vi "WeightingCheck.vi"() -> ()   [LabVIEW 2012]
uses:
  <vilib>/addons/database/Auxilliary.llb/DB Tools Cursor Type.ctl
  <vilib>/addons/database/Connection.llb/DB Tools Open Connec (Path).vi
  <vilib>/Utility/file.llb/Read From Spreadsheet File (string).vi
  <vilib>/addons/database/Connection.llb/Conn Execute.vi
  <vilib>/addons/database/Recordset.llb/Rec Fetch Integer Data (R).vi
  <vilib>/addons/database/Recordset.llb/Rec Destroy - Connection.vi
  <vilib>/Utility/file.llb/Write To Spreadsheet File (string).vi
  <vilib>/addons/database/NI_Database_API.lvlib
panel:
  out "error out":errorcluster
  out "filenames":string[](array[string])
  out "Wrong RC":bool
  out "STD Weight Check":bool
  out "ProdLine":bool
  out "Total Check":bool
  out "Pass Check":bool
  out "data":i32
  in  "Cluster":T1
  out "after substring":string
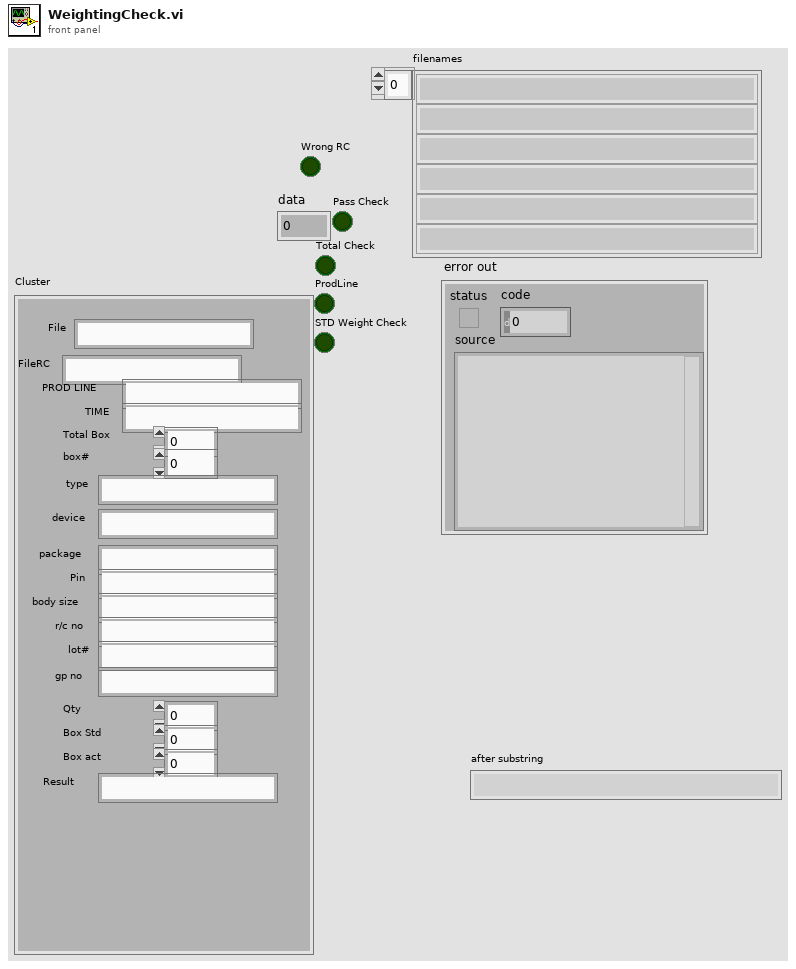
[diagram p1: front panel]
types:
  T1 = cluster{"File":string, "FileRC":string, "PROD LINE ":string, "TIME":string, "Total Box":dbl, "box#":dbl, "type":string, "device":string, "package":string, "Pin ":string, "body size":string, "r/c no":string, "lot#":string, "gp no":string, "Qty":dbl, "Box Std":dbl, "Box act":dbl, "Result":string}
  T2 = typedef "NI_Database_API.lvlib/DB Tools Cursor Type.ctl" = enum16{"forward-only", "keyset", "dynamic", "static"}
  T3 = typedef "NI_Database_API.lvlib/Conn ObjectReference.ctl" = refnum<k1>
  T4 = typedef "NI_Database_API.lvlib/Rec ObjectReference.ctl" = refnum<k1>
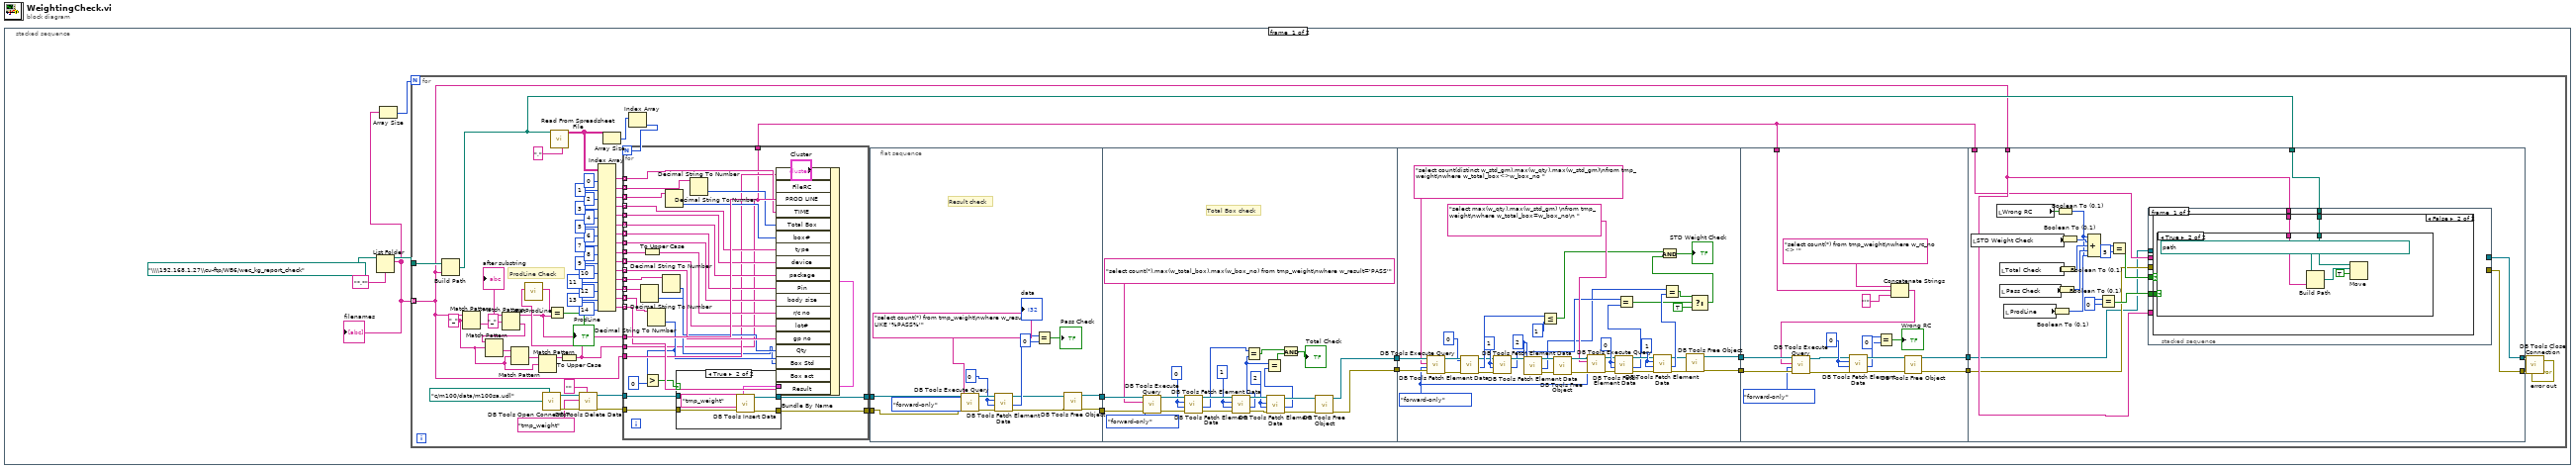
[diagram p0: block diagram]
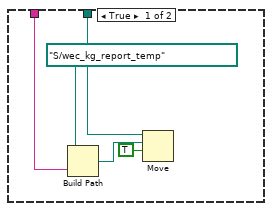
[diagram p2: hidden frame]
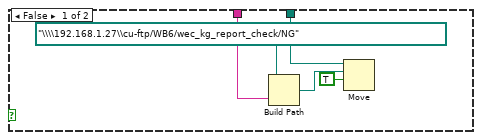
[diagram p3: hidden frame]
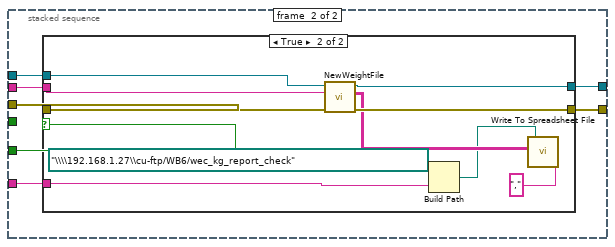
[diagram p4: hidden frame]
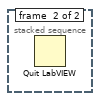
[diagram p7: hidden frame]
diagram:
  n1 = stacked-sequence {
    frame #0 {
      n2 = List Folder(path=path "\\\\192.168.1.27\\cu-ftp/WB6/wec_kg_report_check", pattern="*.*") -> (path out=w3:path, filenames=w1:string[])  [unwired: 2 in, 2 out]
      "filenames" <- w1
      n3 = Array Size(array=w1) -> (size(s)=w2:i32)
      n4 = for {
        N: w2 -> [_]
        tunnel: w3 -> [w56]
        tunnel: w1 -> [w10] mode=indexing
        w51 = "_" ("regular expression")
        # "ProdLine Check"
        n5 = Build Path(base path=w56, name or relative path=w10) -> (appended path=w11:path)
        n6 = Match Pattern(string=w10, regular expression=w51) -> (after substring=w54:string)  [unwired: 1 in, 3 out]
        "after substring" <- w54
        n7 = Match Pattern(string=w54, regular expression="_") -> (before substring=w19:string, after substring=w50:string)  [unwired: 1 in, 2 out]
        n8 = Match Pattern(string=w50, regular expression=w51) -> (after substring=w53:string)  [unwired: 1 in, 3 out]
        n9 = Match Pattern(string=w53, regular expression=w51) -> (after substring=w52:string)  [unwired: 1 in, 3 out]
        n10 = Match Pattern(string=w52, regular expression=w51) -> (before substring=w49:string)  [unwired: 1 in, 3 out]
        n11 = call-poly <vilib>:"DB Tools Open Connection.vi"("connection information"=path "c:/m100/data/m100sa.udl") -> ("error out"=w30:errorcluster, "connection reference"=w31:T3)  [unwired: 7 in]
        n12 = call-poly <vilib>:"Read From Spreadsheet File.vi"("delimiter (\\t)"="," ("delimiter (\\t)"), "file path (dialog if empty)"=w11) -> ("all rows"=w72:string[][])  [unwired: 5 in, 4 out]
        n13 = To Upper Case(1:w49) -> (0:w21:string)
        n14 = call "GetProdLine.vi"("Lotno"=w21) -> ("ProdLine"=w20:string)  [unwired: 10 in]
        n15 = Equal?(x=w20, y=w19) -> (x = y?=→"ProdLine":bool)
        n16 = call <vilib>:"DB Tools Delete Data.vi"("condition"="", "error in (no error)"=w30, "table"="tmp_weight", "connection reference"=w31) -> ("error out"=w28:errorcluster, "connection reference out"=w29:T3)  [unwired: 6 in]
        n17 = Index Array(array=w72, index (col) #1=0 ("disabled index (col)"), index (col) #2=1 ("index (col)"), index (col) #3=2 ("index (col)"), index (col) #4=3 ("index (col)"), index (col) #5=4 ("index (col)"), index (col) #6=5 ("index (col)"), index (col) #7=6 ("index (col)"), index (col) #8=7 ("index (col)"), index (col) #9=8 ("index (col)"), index (col) #10=9 ("index (col)"), index (col) #11=10 ("index (col)"), index (col) #12=11 ("index (col)"), index (col) #13=12 ("index (col)"), index (col) #14=13 ("index (col)"), index (col) #15=14 ("index (col)")) -> (element #1=w64:string[], element #2=w62:string[], element #3=w61:string[], element #4=w60:string[], element #5=w59:string[], element #6=w58:string[], element #7=w57:string[], element #8=w42:string[], element #9=w39:string[], element #10=w38:string[], element #11=w37:string[], element #12=w36:string[], element #13=w35:string[], element #14=w34:string[], element #15=w33:string[])  [unwired: 15 in]
        n18 = Array Size(array=w72) -> (size(s)=w73:i32[])
        n19 = Index Array(array=w73) -> (element=w63:i32)  [unwired: 1 in]
        n20 = for {
          N: w63 -> [_]
          tunnel: w64 -> [w258] mode=indexing
          tunnel: w62 -> [w261] mode=indexing
          tunnel: w61 -> [w256] mode=indexing
          tunnel: w60 -> [w254] mode=indexing
          tunnel: w59 -> [w253] mode=indexing
          tunnel: w58 -> [w252] mode=indexing
          tunnel: w57 -> [w251] mode=indexing
          tunnel: w42 -> [w250] mode=indexing
          tunnel: w39 -> [w262] mode=indexing
          tunnel: w38 -> [w248] mode=indexing
          tunnel: w37 -> [w247] mode=indexing
          tunnel: w36 -> [w246] mode=indexing
          tunnel: w35 -> [w244] mode=indexing
          tunnel: w34 -> [w243] mode=indexing
          tunnel: w33 -> [w242] mode=indexing
          tunnel: w21 -> [w231]
          tunnel: w10 -> [w241]
          tunnel: w19 -> [w259]
          tunnel: w29 -> [w240]
          tunnel: w28 -> [w239]
          tunnel: [w238] -> w25
          tunnel: [w237] -> w24
          tunnel: [w231] -> w7
          n21 = Decimal String To Number(string=w244) -> (number=w232:i32)  [unwired: 2 in, 1 out]
          n22 = To Upper Case(1:w262) -> (0:w249:string)
          n23 = Decimal String To Number(string=w243) -> (number=w235:i32)  [unwired: 2 in, 1 out]
          n24 = Greater?(x=w235, y=0) -> (0:w233:bool)
          n25 = Decimal String To Number(string=w246) -> (number=w245:i32)  [unwired: 2 in, 1 out]
          n26 = Decimal String To Number(string=w256) -> (number=w255:i32)  [unwired: 2 in, 1 out]
          n27 = Decimal String To Number(string=w261) -> (number=w257:i32)  [unwired: 2 in, 1 out]
          n28 = Bundle By Name(cluster="Cluster", "File"=w241, "FileRC"=w231, "PROD LINE"=w259, "TIME"=w258, "Total Box"=w257, "box#"=w255, "type"=w254, "device"=w253, "package"=w252, "Pin"=w251, "body size"=w250, "r/c no"=w249, "lot#"=w248, "gp no"=w247, "Qty"=w245, "Box Std"=w232, "Box act"=w235, "Result"=w242) -> (w236:T1)
          n29 = case shown="True" w233 {
            tunnel: w240 -> [w264 w270]
            tunnel: w239 -> [w263 w269]
            tunnel: [w264 w268] -> w238
            tunnel: [w263 w267] -> w237
            tunnel: w236 -> [_ w266]
            frame False {
            }
            frame True {
              n30 = call <vilib>:"DB Tools Insert Data.vi"("data"=w266, "error in (no error)"=w269, "table"="tmp_weight", "connection reference"=w270) -> ("error out"=w267:errorcluster, "connection reference out"=w268:T3)  [unwired: 6 in]
            }
          }
        }
        n31 = flat-sequence {
          tunnel: w25 -> [w88]
          tunnel: [w78] -> w23
          tunnel: w24 -> [w87]
          tunnel: [w77] -> w22
          tunnel: w23 -> [w111]
          tunnel: w22 -> [w110]
          tunnel: [w107] -> w17
          tunnel: [w106] -> w16
          tunnel: w17 -> [w150]
          tunnel: w16 -> [w149]
          tunnel: [w113] -> w15
          tunnel: [w112] -> w14
          tunnel: w15 -> [w167]
          tunnel: w14 -> [w166]
          tunnel: w7 -> [w163]
          tunnel: [w156] -> w13
          tunnel: [w154] -> w12
          tunnel: w13 -> [w168]
          tunnel: w12 -> [w170]
          tunnel: w11 -> [w175]
          tunnel: w10 -> [w171]
          tunnel: [w173] -> w9
          tunnel: [w172] -> w8
          tunnel: w7 -> [w169]
          frame #0 {
            w82 = 0
            # "Result check"
            n32 = call-poly <vilib>:"DB Tools Execute Query.vi"("error in (no error)"=w87, "cursor type"=DB_Tools_Cursor_Type."forward-only", "SQL query"="select count(*) from tmp_weight\nwhere w_result NOT LIKE '%PASS%'", "connection reference"=w88) -> ("error out"=w86:errorcluster, "recordset reference"=w83:T4)  [unwired: 4 in]
            n33 = call-poly <vilib>:"DB Tools Fetch Element Data.vi"("error in (no error)"=w86, "type"=w82, "column index"=w82, "recordset reference"=w83) -> ("error out"=w75:errorcluster, "data"=w81:i32, "recordset reference out"=w76:T4)  [unwired: 3 in]
            "data" <- w81
            n34 = Equal?(x=w81, y=0) -> (x = y?=→"Pass Check":bool)
            n35 = call-poly <vilib>:"DB Tools Free Object.vi"("error in (no error)"=w75, "recordset reference"=w76) -> ("error out"=w77:errorcluster, "connection reference"=w78:T3)  [unwired: 8 in]
          }
          frame #1 {
            w94 = 2
            w100 = 1
            w103 = 0
            # "Total Box check"
            n36 = call-poly <vilib>:"DB Tools Execute Query.vi"("error in (no error)"=w110, "cursor type"=DB_Tools_Cursor_Type."forward-only", "SQL query"="select count(*),max(w_total_box),max(w_box_no) from tmp_weight\nwhere w_result='PASS'", "connection reference"=w111) -> ("error out"=w108:errorcluster, "recordset reference"=w109:T4)  [unwired: 4 in]
            n37 = call-poly <vilib>:"DB Tools Fetch Element Data.vi"("error in (no error)"=w108, "type"=w103, "column index"=w103, "recordset reference"=w109) -> ("error out"=w101:errorcluster, "data"=w99:i32, "recordset reference out"=w102:T4)  [unwired: 3 in]
            n38 = call-poly <vilib>:"DB Tools Fetch Element Data.vi"("error in (no error)"=w101, "type"=w100, "column index"=w100, "recordset reference"=w102) -> ("error out"=w96:errorcluster, "data"=w93:i32, "recordset reference out"=w98:T4)  [unwired: 3 in]
            n39 = Equal?(x=w99, y=w93) -> (x = y?=w90:bool)
            n40 = call-poly <vilib>:"DB Tools Fetch Element Data.vi"("error in (no error)"=w96, "type"=w94, "column index"=w94, "recordset reference"=w98) -> ("error out"=w95:errorcluster, "data"=w92:i32, "recordset reference out"=w97:T4)  [unwired: 3 in]
            n41 = Equal?(x=w93, y=w92) -> (x = y?=w91:bool)
            n42 = And(x=w90, y=w91) -> (x .and. y?=→"Total Check":bool)
            n43 = call-poly <vilib>:"DB Tools Free Object.vi"("error in (no error)"=w95, "recordset reference"=w97) -> ("error out"=w106:errorcluster, "connection reference"=w107:T3)  [unwired: 8 in]
          }
          frame #2 {
            w134 = 1
            w135 = 0
            w138 = 2
            w142 = 1
            w145 = 0
            w127 = DB_Tools_Cursor_Type."forward-only" ("cursor type")
            n44 = call-poly <vilib>:"DB Tools Execute Query.vi"("error in (no error)"=w149, "cursor type"=w127, "SQL query"="select count(distinct w_std_gm),max(w_qty),max(w_std_gm)\nfrom tmp_weight\nwhere w_total_box<>w_box_no ", "connection reference"=w150) -> ("error out"=w147:errorcluster, "recordset reference"=w148:T4)  [unwired: 4 in]
            n45 = call-poly <vilib>:"DB Tools Fetch Element Data.vi"("error in (no error)"=w147, "type"=w145, "column index"=w145, "recordset reference"=w148) -> ("error out"=w140:errorcluster, "data"=w144:i32, "recordset reference out"=w141:T4)  [unwired: 3 in]
            n46 = call-poly <vilib>:"DB Tools Fetch Element Data.vi"("error in (no error)"=w140, "type"=w142, "column index"=w142, "recordset reference"=w141) -> ("data"=w125:i32, "recordset reference out"=w139:T4)  [unwired: 3 in, 1 out]
            n47 = call-poly <vilib>:"DB Tools Fetch Element Data.vi"("type"=w138, "column index"=w138, "recordset reference"=w139) -> ("error out"=w136:errorcluster, "data"=w123:i32, "recordset reference out"=w137:T4)  [unwired: 4 in]
            n48 = Less Or Equal?(x=w144, y=1) -> (x <= y?=w118:bool)
            n49 = call-poly <vilib>:"DB Tools Free Object.vi"("error in (no error)"=w136, "recordset reference"=w137) -> ("error out"=w128:errorcluster, "connection reference"=w129:T3)  [unwired: 8 in]
            n50 = call-poly <vilib>:"DB Tools Execute Query.vi"("error in (no error)"=w128, "cursor type"=w127, "SQL query"="select max(w_qty),max(w_std_gm) \nfrom tmp_weight\nwhere w_total_box=w_box_no\n ", "connection reference"=w129) -> ("error out"=w130:errorcluster, "recordset reference"=w131:T4)  [unwired: 4 in]
            n51 = call-poly <vilib>:"DB Tools Fetch Element Data.vi"("error in (no error)"=w130, "type"=w135, "column index"=w135, "recordset reference"=w131) -> ("error out"=w132:errorcluster, "data"=w124:i32, "recordset reference out"=w133:T4)  [unwired: 3 in]
            n52 = Equal?(x=w125, y=w124) -> (x = y?=w121:bool)
            n53 = call-poly <vilib>:"DB Tools Fetch Element Data.vi"("error in (no error)"=w132, "type"=w134, "column index"=w134, "recordset reference"=w133) -> ("error out"=w114:errorcluster, "data"=w122:i32, "recordset reference out"=w115:T4)  [unwired: 3 in]
            n54 = Equal?(x=w123, y=w122) -> (x = y?=w120:bool)
            n55 = call-poly <vilib>:"DB Tools Free Object.vi"("error in (no error)"=w114, "recordset reference"=w115) -> ("error out"=w112:errorcluster, "connection reference"=w113:T3)  [unwired: 8 in]
            n56 = Select(t=w120, s=w121, f=TRUE) -> (s? t:f=w117:bool)
            n57 = And(x=w118, y=w117) -> (x .and. y?=→"STD Weight Check":bool)
          }
          frame #3 {
            w160 = 0
            n58 = Concatenate Strings("select count(*) from tmp_weight\nwhere w_rc_no <> '", w163, "'") -> (w161:string)
            n59 = call-poly <vilib>:"DB Tools Execute Query.vi"("error in (no error)"=w166, "cursor type"=DB_Tools_Cursor_Type."forward-only", "SQL query"=w161, "connection reference"=w167) -> ("error out"=w158:errorcluster, "recordset reference"=w159:T4)  [unwired: 4 in]
            n60 = call-poly <vilib>:"DB Tools Fetch Element Data.vi"("error in (no error)"=w158, "type"=w160, "column index"=w160, "recordset reference"=w159) -> ("error out"=w155:errorcluster, "data"=w153:i32, "recordset reference out"=w157:T4)  [unwired: 3 in]
            n61 = Equal?(x=w153, y=0) -> (x = y?=→"Wrong RC":bool)
            n62 = call-poly <vilib>:"DB Tools Free Object.vi"("error in (no error)"=w155, "recordset reference"=w157) -> ("error out"=w154:errorcluster, "connection reference"=w156:T3)  [unwired: 8 in]
          }
          frame #4 {
            n63 = local read "STD Weight Check"() -> (w188:bool)
            n64 = local read "Wrong RC"() -> (w189:bool)
            n65 = local read "Total Check"() -> (w187:bool)
            n66 = local read "Pass Check"() -> (w186:bool)
            n67 = local read "ProdLine"() -> (w185:bool)
            n68 = Boolean To (0,1)(Boolean=w185) -> (0, 1=w181:i16)
            n69 = Boolean To (0,1)(Boolean=w189) -> (0, 1=w177:i16)
            n70 = Boolean To (0,1)(Boolean=w186) -> (0, 1=w182:i16)
            n71 = Boolean To (0,1)(Boolean=w187) -> (0, 1=w183:i16)
            n72 = Boolean To (0,1)(Boolean=w188) -> (0, 1=w184:i16)
            n73 = Compound Arithmetic op=ADD(w177, w184, w183, w182, w181) -> (w180:i16)
            n74 = Equal?(x=w177, y=i16 0) -> (x = y?=w174:bool)
            n75 = Equal?(x=w180, y=i16 5) -> (x = y?=w178:bool)
            n76 = stacked-sequence {
              tunnel: w178 -> [w193 _]
              tunnel: w171 -> [w192 _]
              tunnel: w175 -> [w191 _]
              tunnel: w174 -> [w190 w216]
              tunnel: [_ w218] -> w173
              tunnel: [_ w217] -> w172
              tunnel: w171 -> [_ w215]
              tunnel: w170 -> [_ w214]
              tunnel: w169 -> [_ w213]
              tunnel: w168 -> [_ w212]
              frame #0 {
                n77 = case shown="False" w193 {
                  tunnel: w191 -> [w198 w201]
                  tunnel: w192 -> [w195 w200]
                  tunnel: w190 -> [_ w199]
                  frame True {
                    n78 = Build Path(base path=path "S:/wec_kg_report_temp", name or relative path=w195) -> (appended path=w197:path)
                    n79 = Move(source path=w198, 9:TRUE ("overwrite (F)"), 10:w197) -> ()  [unwired: 2 in, 3 out]
                  }
                  frame False {
                    n80 = case shown="True" w199 {
                      tunnel: w201 -> [w206 w211]
                      tunnel: w200 -> [w203 w208]
                      frame False {
                        n81 = Build Path(base path=path "\\\\192.168.1.27\\cu-ftp/WB6/wec_kg_report_check/NG", name or relative path=w203) -> (appended path=w205:path)
                        n82 = Move(source path=w206, 9:TRUE ("overwrite (F)"), 10:w205) -> ()  [unwired: 2 in, 3 out]
                      }
                      frame True {
                        n83 = Build Path(base path=path "\\\\192.168.1.27\\cu-ftp/WB6/wec_kg_report_check/修正前", name or relative path=w208) -> (appended path=w210:path)
                        n84 = Move(source path=w211, 9:TRUE ("overwrite (F)"), 10:w210) -> ()  [unwired: 2 in, 3 out]
                      }
                    }
                  }
                }
              }
              frame #1 {
                n85 = case shown="True" w216 {
                  tunnel: w212 -> [w220 w230]
                  tunnel: w214 -> [w219 w229]
                  tunnel: [w220 w228] -> w218
                  tunnel: [w219 w227] -> w217
                  tunnel: w215 -> [_ w226]
                  tunnel: w213 -> [_ w225]
                  frame False {
                  }
                  frame True {
                    n86 = call "NewWeightFile.vi"("error in (no error)"=w229, "RC No"=w225, "connection reference"=w230) -> ("error out"=w227:errorcluster, "Array"=w223:string[][], "connection reference out"=w228:T3)  [unwired: 6 in]
                    n87 = Build Path(base path=path "\\\\192.168.1.27\\cu-ftp/WB6/wec_kg_report_check", name or relative path=w226) -> (appended path=w222:path)
                    n88 = call-poly <vilib>:"Write To Spreadsheet File.vi"("delimiter (\\t)"="," ("delimiter (\\t)"), "2D data"=w223, "file path (dialog if empty)"=w222) -> ()  [unwired: 5 in, 1 out]
                  }
                }
              }
            }
          }
        }
        n89 = call <vilib>:"DB Tools Close Connection.vi"("error in (no error)"=w8, "connection reference"=w9) -> ("error out"=→"error out":errorcluster)  [unwired: 5 in]
      }
    }
    frame #1 {
      n90 = Quit LabVIEW() -> ()  [unwired: 1 in]
    }
  }
